vi "Response Completeness.vi"(8 "error in (no error)":errorcluster, 10 "Bytes at Port":u32, 11 "Response Buffer":string) -> (0 "error out":errorcluster, 3 "Response Complete?":bool)   [LabVIEW 2018, in "ESM303.lvlib" / "ESM303.lvclass"]
uses:
  ESM303.lvclass
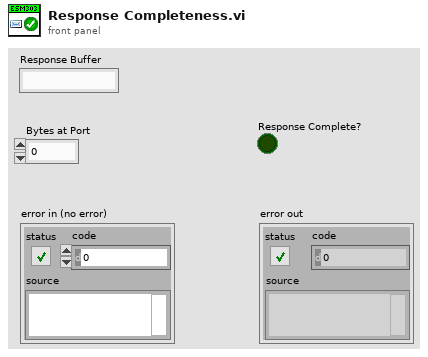
[diagram p1: front panel]
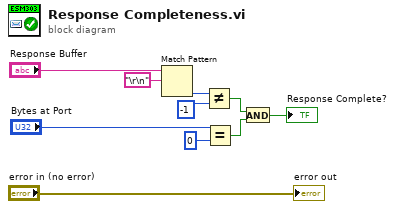
[diagram p0: block diagram]
diagram:
  n1 = Match Pattern(string="Response Buffer", regular expression="\r\n") -> (offset past match=w8:i32)  [unwired: 1 in, 3 out]
  n2 = Not Equal?(x=w8, y=-1) -> (x != y?=w5:bool)
  n3 = Equal?(x="Bytes at Port", y=u32 0) -> (x = y?=w6:bool)
  n4 = And(x=w5, y=w6) -> (x .and. y?=→"Response Complete?":bool)
  "error out" <- "error in (no error)"
